vi "Bind DBL parameter.vi"(4 "error in (no error)":errorcluster, 6 "Parameter":dbl format="%.2f", 7 "Statement Refnum":T1) -> (0 "error out":errorcluster, 3 "Statement Refnum":T1)   [LabVIEW 2011]
doc: "Charge le paramètre de type réel double (DBL) dans la pile"
uses:
  SQL Controls/Statement Refnum.ctl
  Odbc32.dll
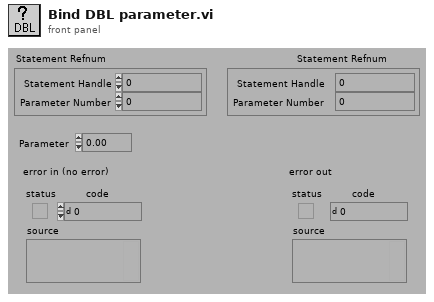
[diagram p1: front panel]
types:
  T1 = typedef "Statement Refnum.ctl" = cluster{"Statement Handle":i32, "Parameter Number":u16}
  T2 = enum16{"NOPE", "SQL_HANDLE_ENV", "SQL_HANDLE_DBC", "SQL_HANDLE_STMT", "SQL_HANDLE_DESC"}
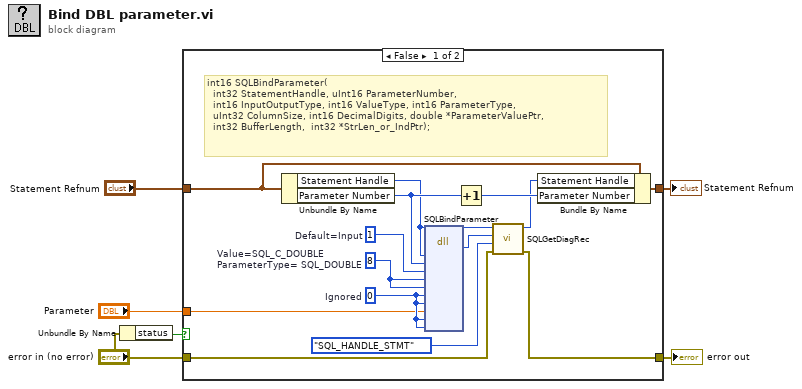
[diagram p0: block diagram]
diagram:
  n1 = Unbundle By Name("error in (no error)") -> ("status"=w1:bool)
  n2 = case shown="False" w1 {
    tunnel: "Statement Refnum" -> [w18 w21]
    tunnel: [w17 w21] -> w5
    tunnel: "Parameter" -> [w13 _]
    tunnel: "error in (no error)" -> [w10 w22]
    tunnel: [w9 w22] -> w3
    frame False {
      w12 = i16 8  # Value=SQL_C_DOUBLE ParameterType= SQL_DOUBLE
      w20 = 0  # Ignored
      w15 = i16 1  # Default=Input
      # "int16 SQLBindParameter(\n  int32 StatementHandle, uInt16 ParameterNumber, \n  int16 InputOutputType, int16 ValueType, int16 ParameterType, \n  uInt32 ColumnSize, int16 DecimalDigits, double *ParameterValuePtr,\n  int32 BufferLength,  int32 *StrLen_or_IndPtr);"
      n3 = Unbundle By Name(w18) -> ("Statement Handle"=w11:i32, "Parameter Number"=w16:u16)
      n4 = dll-call lib="Odbc32.dll" fn="SQLBindParameter"("StatementHandle"=w11, "ParameterNumber"=w16, "InputOutputType"=w15, "ValueType"=w12, "ParameterType"=w12, "ColumnSize"=w20, "DecimalDigits"=w20, "ParameterValuePtr"=w13, "BufferLength"=w20, "StrLen_or_IndPtr"=w20) -> (w19:i16)  [unwired: 11 in, 4 out]
      n5 = Increment(x=w16) -> (x+1=w14:u16)
      n6 = call "SQLGetDiagRec.vi"("error in (no error)"=w10, "HandleType"=T2."SQL_HANDLE_STMT", "Status (SQL_SUCCESS=0)"=w19, "Input Handle"=w11) -> ("error out"=w9:errorcluster, "Output Handle"=w8:i32)  [unwired: 2 out]
      n7 = Bundle By Name(cluster=w18, "Statement Handle"=w8, "Parameter Number"=w14) -> (w17:T1)
    }
    frame True {
    }
  }
  "Statement Refnum" <- w5
  "error out" <- w3
